vi "PathPlanner_IdealStartingState_GetAll.vi"(11 "GoalEndState":T2={"VelocityMPS"=0.0, "Rotation"={"VALUE"=0.0, "COS"=1.0, "SIN"=0.0}} {"Rotation"."SIN" format="%13.4f"; "Rotation"."COS" format="%13.4f"; "Rotation"."VALUE" format="%13.4f"}) -> (1 "Rotation":T1={"VALUE"=0.0, "COS"=1.0, "SIN"=0.0} {"SIN" format="%13.4f"; "COS" format="%13.4f"; "VALUE" format="%13.4f"}, 3 "VelocityMPS":dbl)   [LabVIEW 2019, in "PathPlanner24.lvlib"]
doc: "Get the ideal starting state velocity and end rotation\n \n\nInputs: \n -- IdealStartingState - cluster - definition data structure\n\nOutputs:\n -- Ideal starting velocity (M/S)\n -- Ideal starting rotation"
uses:
  TypeDef/PathPlannerGoalEndState.ctl
  <vilib>/Rock Robotics/WPI/ThirdParty/JAS_Junk/TrajLib/TypeDef/ROTATION2D.ctl
  PathPlanner24.lvlib
  <vilib>/Rock Robotics/WPI/ThirdParty/JAS_Junk/TrajLib/Trajectory_Library.lvlib
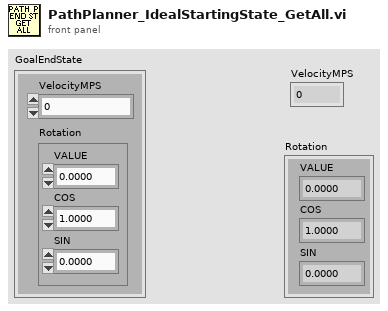
[diagram p1: front panel]
types:
  T1 = typedef "Trajectory_Library.lvlib/ROTATION2D.ctl" = cluster{"VALUE":dbl, "COS":dbl, "SIN":dbl}
  T2 = typedef "PathPlanner24.lvlib/PathPlannerGoalEndState.ctl" = cluster{"VelocityMPS":dbl, "Rotation":T1}
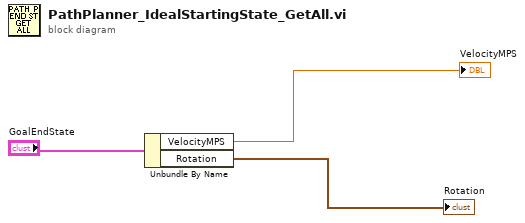
[diagram p0: block diagram]
diagram:
  n1 = Unbundle By Name("GoalEndState") -> ("VelocityMPS"=→"VelocityMPS":dbl, "Rotation"=→"Rotation":T1)
